vi "ダミーデータ変換.vi"(10 "signal out":waveform(dbl), 11 "signal out 2":waveform(dbl) caption="signal out") -> (1 "パワースペクトル":cluster{"f0":dbl, "df":dbl, "magnitude":dbl[]}[](array[cluster]), 2 "Wave[]":T1[](array[typedef]), 3 "Chart[]":dbl[][](array[numeric]))   [LabVIEW 2014]
uses:
  View/GraphSetting/TypeDef/WaveData.ctl
  <vilib>/measure/maspectr.llb/FFT Power Spectrum and PSD for 1 Chan.vi
  <vilib>/measure/NI_MAPro.lvlib
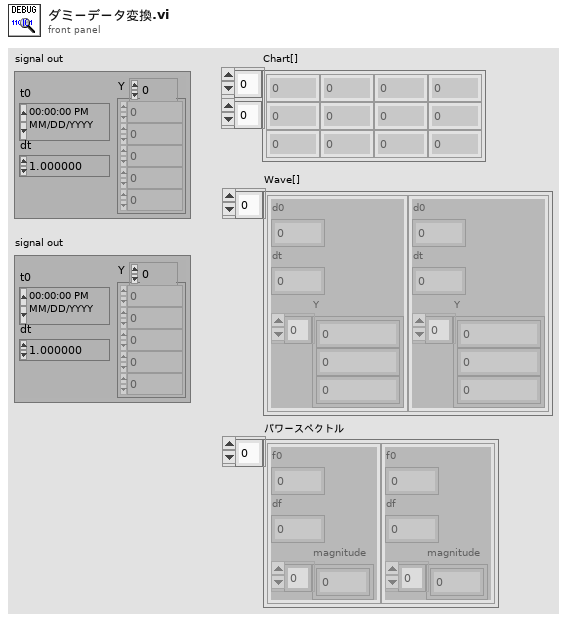
[diagram p1: front panel]
types:
  T1 = typedef "WaveData.ctl" = cluster{"d0":dbl, "dt":dbl, "Y":dbl[]}
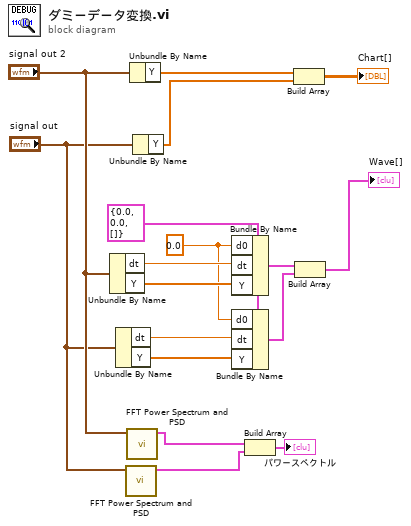
[diagram p0: block diagram]
diagram:
  w10 = 0.0 ("Fs")
  w9 = T1 {"d0"=0.0, "dt"=0.0, "Y"=[]} ("波形データ")
  n1 = Unbundle By Name("signal out 2") -> ("dt"=w11:dbl, "Y"=w12:dbl[])
  n2 = Unbundle By Name("signal out") -> ("dt"=w13:dbl, "Y"=w14:dbl[])
  n3 = call-poly <vilib>:"FFT Power Spectrum and PSD.vi"("time signal"="signal out") -> ("Power Spectrum / PSD"=w5:cluster{"f0":dbl, "df":dbl, "magnitude":dbl[]})  [unwired: 7 in, 3 out]
  n4 = call-poly <vilib>:"FFT Power Spectrum and PSD.vi"("time signal"="signal out 2") -> ("Power Spectrum / PSD"=w4:cluster{"f0":dbl, "df":dbl, "magnitude":dbl[]})  [unwired: 7 in, 3 out]
  n5 = Unbundle By Name("signal out 2") -> ("Y"=w6:dbl[])
  n6 = Unbundle By Name("signal out") -> ("Y"=w7:dbl[])
  n7 = Bundle By Name(cluster=w9, "d0"=w10, "dt"=w11, "Y"=w12) -> (w15:T1)
  n8 = Bundle By Name(cluster=w9, "d0"=w10, "dt"=w13, "Y"=w14) -> (w16:T1)
  n9 = Build Array(w4, w5) -> (→"パワースペクトル":cluster{"f0":dbl, "df":dbl, "magnitude":dbl[]}[])
  n10 = Build Array(w6, w7) -> (→"Chart[]":dbl[][])
  n11 = Build Array(w15, w16) -> (→"Wave[]":T1[])
